vi "Self-Test.vi"(8 "error in (no error)":errorcluster, 11 "VISA resource name":refnum<visa-resource-name>) -> (0 "error out":errorcluster, 1 "self-test response":string, 2 "self-test error":bool, 3 "VISA resource name out":refnum<visa-resource-name>)   [LabVIEW 2009, in "Fluke 8840.lvlib"]
doc: "This VI causes the instrument to perform a self-test and returns the results. A boolean indicates if the instrument passed self-test, and string contains the instruments reponse."
uses:
  Fluke 8840.lvlib
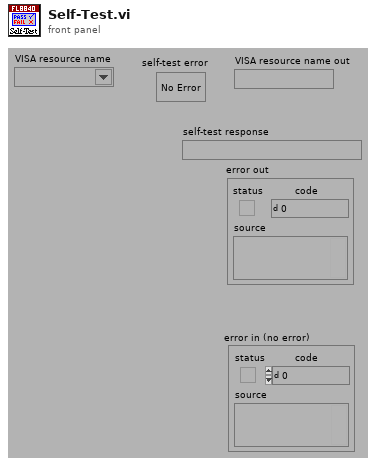
[diagram p1: front panel]
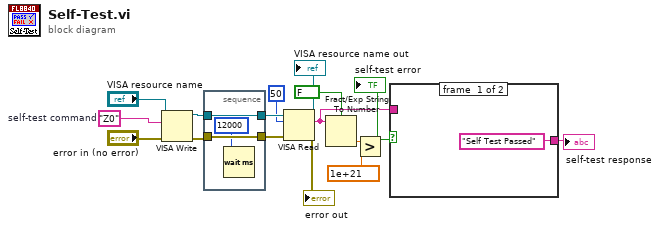
[diagram p0: block diagram]
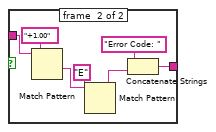
[diagram p2: hidden frame]
diagram:
  w16 = "Z0"  # self-test command
  n1 = VISA Write(VISA resource name="VISA resource name", write buffer=w16, error in (no error)="error in (no error)") -> (VISA resource name out=w13:refnum<visa-resource-name>, error out=w12:errorcluster)  [unwired: 1 out]
  n2 = stacked-sequence {
    tunnel: w13 -> [w18]
    tunnel: w12 -> [w19]
    tunnel: [w19] -> w10
    tunnel: [w18] -> w11
    frame #0 {
      n3 = Wait (ms)(milliseconds to wait=u32 12000) -> ()  [unwired: 1 out]
    }
  }
  n4 = VISA Read(VISA resource name=w11, byte count=u32 50, error in (no error)=w10) -> (VISA resource name out=→"VISA resource name out":refnum<visa-resource-name>, read buffer=w2:string, error out=→"error out":errorcluster)  [unwired: 1 out]
  n5 = Fract/Exp String To Number(use system decimal point (T)=FALSE, string=w2) -> (number=w7:dbl)  [unwired: 3 out]
  n6 = Greater?(x=w7, y=1e+21) -> (0:w5:bool)
  "self-test error" <- w5
  n7 = case shown="True" w5 {
    tunnel: w2 -> [_ w26]
    tunnel: ["Self Test Passed" w21] -> w3
    frame #0 {
    }
    frame #1 {
      n8 = Match Pattern(string=w26, regular expression="+1.00") -> (after substring=w25:string)  [unwired: 4 out]
      n9 = Match Pattern(string=w25, regular expression="E") -> (before substring=w23:string)  [unwired: 4 out]
      n10 = Concatenate Strings("Error Code: ", w23) -> (w21:string)
    }
  }
  "self-test response" <- w3
